vi "tt20panel_DO_connect.vi"(8 "error in (no error)":errorcluster, 9 "tt20_settings":T1, 10 "tt20_events":T3, 11 "tt20panel in":refnum<class "tt20panel.lvclass">) -> (0 "error out":errorcluster, 3 "tt20panel out":refnum<class "tt20panel.lvclass">)   [LabVIEW 2015, in "tt20panel.lvclass"]
uses:
  tt20panel.lvclass
  tt20_event_tdef.ctl
  tt20_class/tt20_hardware_info_tdef.ctl
  tt20_acq_mode_tdef.ctl
  tt20_class/tt20.lvclass
  tt20_class/tt20.lvclass/tt20.ctl
  UI/panel_class/panel.lvclass
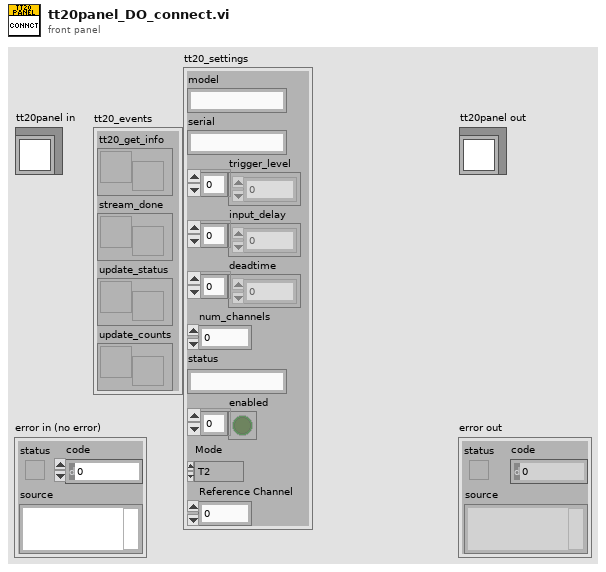
[diagram p1: front panel]
types:
  T1 = typedef "tt20_hardware_info_tdef.ctl" = cluster{"model":string, "serial":string, "trigger_level":dbl[], "input_delay":i64[], "deadtime":i64[], "num_channels":u32, "status":string, "enabled":bool[], "Mode":T2, "Reference Channel":u8}
  T2 = typedef "tt20_acq_mode_tdef.ctl" = enum16{"T2", "T3"}
  T3 = typedef "tt20_event_tdef.ctl" = cluster{"tt20_get_info":refnum<user-event>, "stream_done":refnum<user-event>, "update_status":refnum<user-event>, "update_counts":refnum<user-event>}
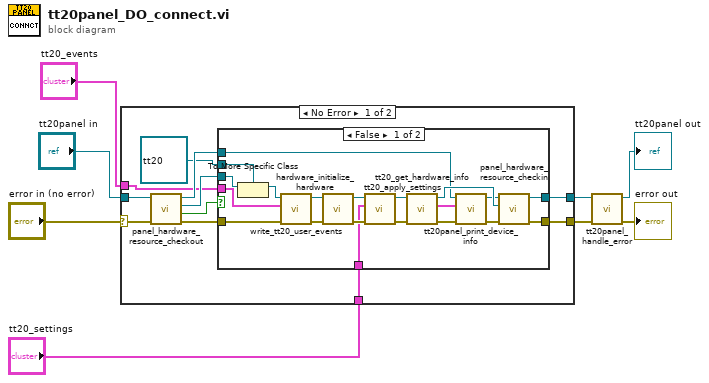
[diagram p0: block diagram]
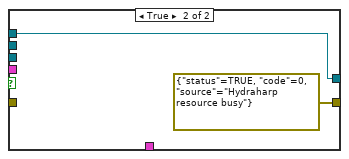
[diagram p2: hidden frame]
diagram:
  n1 = case shown="No Error" "error in (no error)" {
    selector: "error in (no error)" -> [w18 w43]
    tunnel: [w15 w43] -> w5
    tunnel: [w12 w42] -> w3
    tunnel: "tt20panel in" -> [w19 w42]
    tunnel: "tt20_events" -> [w10 _]
    tunnel: "tt20_settings" -> [w9 _]
    frame No Error {
      n2 = call "panel_hardware_resource_checkout.vi"("error in (no error)"=w18, "panel in"=w19) -> ("error out"=w16:errorcluster, "timed out?"=w17:bool, "hardware.lvclass"=w13:refnum<class "hardware.lvclass">, "panel out"=w14:refnum<class "tt20panel.lvclass">)  [unwired: 6 in]
      n3 = case shown="False" w17 {
        tunnel: w16 -> [w34 _]
        tunnel: [w37 errorcluster {"status"=TRUE, "code"=0, "source"="Hydraharp resource busy"} ("error out")] -> w15
        tunnel: w14 -> [w26 w40]
        tunnel: w13 -> [w38 _]
        tunnel: refnum<class "tt20.lvclass"> refnum ("tt20.lvclass") -> [w39 _]
        tunnel: [w36 w40] -> w12
        tunnel: w10 -> [w30 _]
        tunnel: w9 -> [w20 _]
        frame False {
          n4 = To More Specific Class(target class=w39, reference=w38) -> (specific class reference=w32:refnum<class "tt20.lvclass">)  [unwired: 1 in, 1 out]
          n5 = call "write_tt20_user_events.vi"("error in (no error)"=w34, "tt20_events"=w30, "tt20 in"=w32) -> ("error out"=w33:errorcluster, "tt20 out"=w31:refnum<class "tt20.lvclass">)  [unwired: 7 in]
          n6 = call-dynamic "hardware_initialize_hardware.vi"("error in (no error)"=w33, "tt20 in"=w31) -> ("error out"=w24:errorcluster, "tt20 out"=w22:refnum<class "tt20.lvclass">)  [unwired: 8 in]
          n7 = call "tt20_apply_settings.vi"("error in (no error)"=w24, "tt20_info"=w20, "tt20 in"=w22) -> ("error out"=w23:errorcluster, "tt20 out"=w21:refnum<class "tt20.lvclass">)  [unwired: 7 in]
          n8 = call "tt20_get_hardware_info.vi"("error in (no error)"=w23, "tt20 in"=w21) -> ("error out"=w29:errorcluster, "tt20_info"=w27:T1, "tt20 out"=w35:refnum<class "tt20.lvclass">)  [unwired: 7 in]
          n9 = call "tt20panel_print_device_info.vi"("error in (no error)"=w29, "tt20_info"=w27, "tt20panel in"=w26) -> ("error out"=w28:errorcluster, "tt20panel out"=w25:refnum<class "tt20panel.lvclass">)  [unwired: 7 in]
          n10 = call "panel_hardware_resource_checkin.vi"("error in (no error)"=w28, "hardware.lvclass"=w35, "panel in"=w25) -> ("error out"=w37:errorcluster, "panel out"=w36:refnum<class "tt20panel.lvclass">)  [unwired: 7 in]
        }
        frame True {
        }
      }
    }
    frame Error {
    }
  }
  n11 = call "tt20panel_handle_error.vi"("error in (no error)"=w5, "tt20panel in"=w3) -> ("error out"=→"error out":errorcluster, "tt20panel out"=→"tt20panel out":refnum<class "tt20panel.lvclass">)  [unwired: 8 in]
